vi "Get User Interface VI.vi"(8 "error in (no error)":errorcluster, 11 "Transfer User Interface in":refnum<class "Transfer User Interface.lvclass">) -> (0 "error out":errorcluster, 2 "user interface vi":refnum<vi>, 3 "Transfer User Interface out":refnum<class "Transfer User Interface.lvclass">)   [LabVIEW 2017, in "PXImc.lvlib" / "Transfer User Interface.lvclass"]
uses:
  Transfer User Interface.lvclass
  User Interface.vi
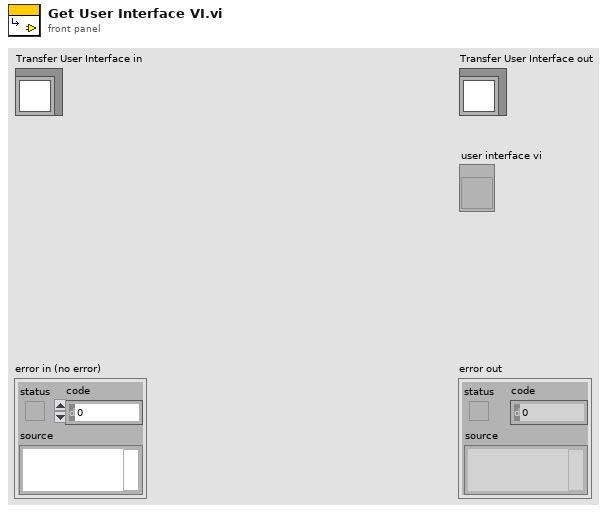
[diagram p1: front panel]
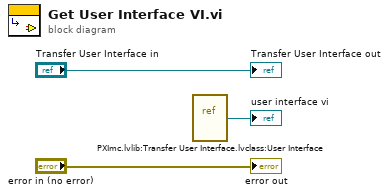
[diagram p0: block diagram]
diagram:
  n1 = vi-ref "PXImc.lvlib:Transfer User Interface.lvclass:User Interface.vi"() -> (→"user interface vi":refnum<vi>)
  "error out" <- "error in (no error)"
  "Transfer User Interface out" <- "Transfer User Interface in"
